vi "WriteToFifo-1.vi"(6 "AXI_STR_RXD_tkeep":fxp<+,4,4>=15.0, 8 "error in (no error)":errorcluster, 9 "Timeout (ms)":i32=5000, 10 "Data":u32[](array[numeric]), 11 "FpgaInterface in":refnum<class "FpgaInterface.lvclass">) -> (0 "error out":errorcluster, 3 "FpgaInterface out":refnum<class "FpgaInterface.lvclass">)   [LabVIEW 2017, in "FpgaInterface.lvclass"]
uses:
  FpgaInterface.lvclass
  FpgaInterface.lvclass/FpgaInterface.ctl
  <vilib>/Utility/error.llb/Error Cluster From Error Code.vi
  <vilib>/rvi/errors/niLvFpgaAdjustHostInterfaceError.vi
  <vilib>/rvi/interface/nirviReadWriteControl/nirviReadWriteControl.xnode
  <vilib>/rvi/interface/nirviMethod/nirviMethod.xnode
  <vilib>/FPGAPlugInAG/Dynamic/niLvFpga_WriteFifo_Dynamic.vi
  <vilib>/rvi/errors/niLvFpgaMergeErrorWithErrorCode.vi
  NiFpgaLv.dll
  <vilib>/rvi/interface/Simulation/niFpgaSimulationCallBeginRW.vi
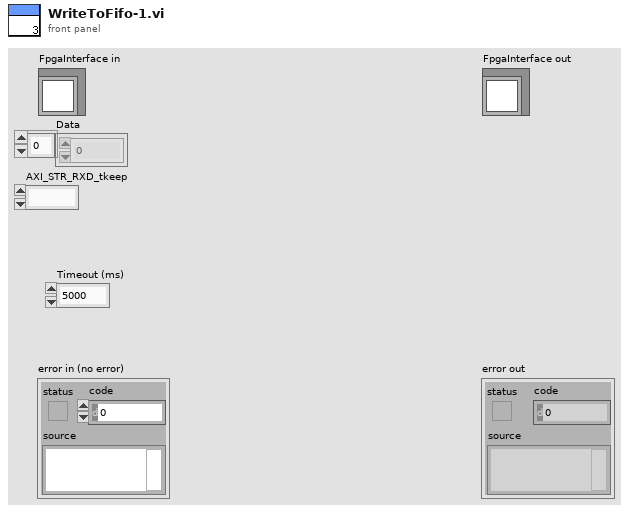
[diagram p1: front panel]
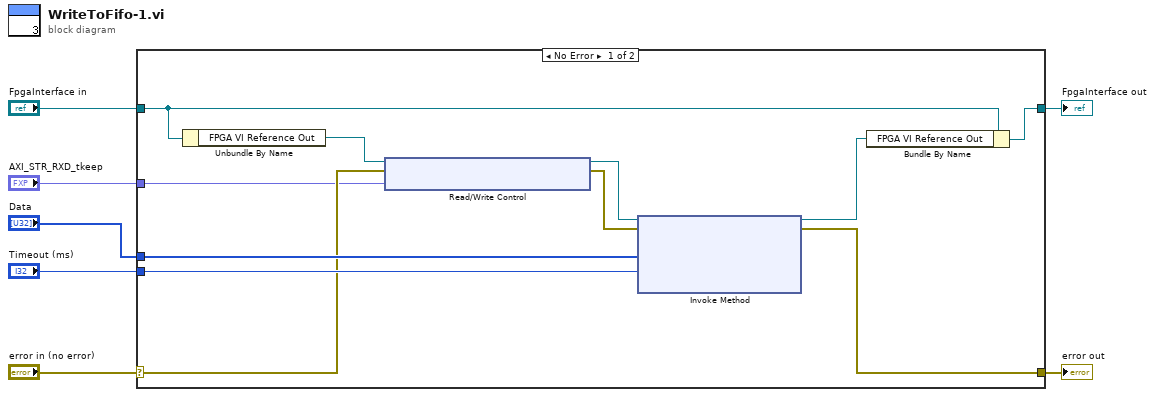
[diagram p0: block diagram]
diagram:
  n1 = case shown="No Error" "error in (no error)" {
    selector: "error in (no error)" -> [w11 w20]
    tunnel: [w16 w20] -> w6
    tunnel: [w13 w19] -> w4
    tunnel: "FpgaInterface in" -> [w14 w19]
    tunnel: "Timeout (ms)" -> [w18 _]
    tunnel: "Data" -> [w17 _]
    tunnel: "AXI_STR_RXD_tkeep" -> [w8 _]
    frame No Error {
      n2 = Unbundle By Name(w14) -> ("FPGA VI Reference Out"=w12:refnum<k20>)
      n3 = xnode "Read/Write Control"("FPGA VI Reference In"=w12, "error in"=w11, "d_microblaze_i\\AXI_STR_RXD_tkeep"=w8) -> ("FPGA VI Reference Out"=w9:refnum<k20>, "error out"=w10:errorcluster)
      n4 = xnode "Invoke Method"("FPGA VI Reference In"=w9, "error in"=w10, "Data"=w17, "Timeout (ms)"=w18) -> ("FPGA VI Reference Out"=w15:refnum<k20>, "error out"=w16:errorcluster)  [unwired: 1 out]
      n5 = Bundle By Name(cluster=w14, "FPGA VI Reference Out"=w15) -> (w13:refnum<class "FpgaInterface.lvclass">)
    }
    frame Error {
    }
  }
  "error out" <- w6
  "FpgaInterface out" <- w4
